vi "EXA shm log Event Applied Settings Match Start LV.vi"(8 "error in (no error)":errorcluster, 11 "logevent_AppliedSettingsMatchStart_Ctl":T1) -> (0 "error out":errorcluster, 2 "function return":i32, 3 "logevent_AppliedSettingsMatchStart_Ctl out":T1)   [LabVIEW 2016, in "SALLV_EXA.lvlib"]
doc: "int EXA_shm_logEvent_AppliedSettingsMatchStartLV(EXA_logevent_AppliedSettingsMatchStartLV *logevent_AppliedSettingsMatchStart_Ctl );"
uses:
  SALLV_EXA.lvlib
  SALLV_EXA.so
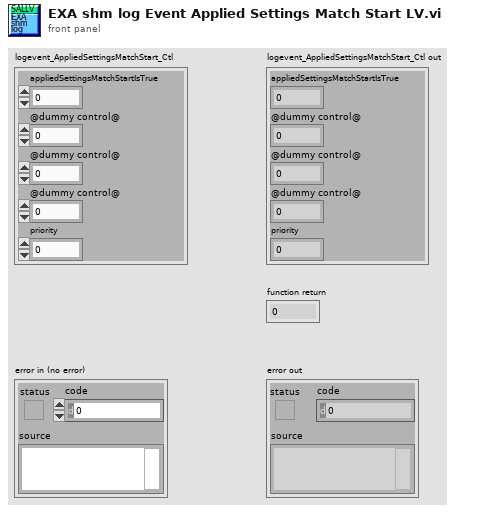
[diagram p1: front panel]
types:
  T1 = cluster{"appliedSettingsMatchStartIsTrue":u8, "@dummy control@":i8, "@dummy control@":i8, "@dummy control@":i8, "priority":i32}
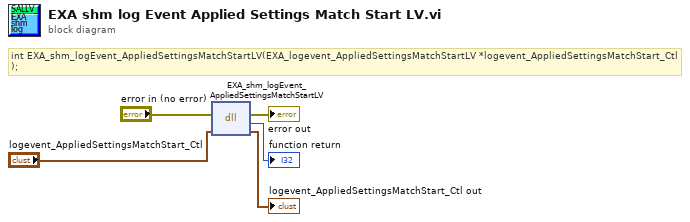
[diagram p0: block diagram]
diagram:
  # "int EXA_shm_logEvent_AppliedSettingsMatchStartLV(EXA_logevent_AppliedSettingsMatchStartLV *logevent_AppliedSettingsMatchStart_Ctl );"
  n1 = dll-call lib="home/plotz/SALLV_EXA/SALLV_EXA.*" fn="EXA_shm_logEvent_AppliedSettingsMatchStartLV"(error in="error in (no error)", "logevent_AppliedSettingsMatchStart_Ctl"="logevent_AppliedSettingsMatchStart_Ctl") -> (error out=→"error out":errorcluster, →"function return":i32, "logevent_AppliedSettingsMatchStart_Ctl"=→"logevent_AppliedSettingsMatchStart_Ctl out":T1)  [unwired: 2 in, 1 out]
